vi "Get List of Names.vi"(8 "error in (no error)":errorcluster, 11 "Kasli in":refnum<class "Kasli.lvclass">) -> (0 "error out":errorcluster, 1 "List of IPs":string[](array[string]), 2 "List of Names":string[](array[string]), 3 "Kasli out":refnum<class "Kasli.lvclass">)   [LabVIEW 2020, in "Kasli Wrapper 2.0.lvlib" / "Kasli.lvclass"]
uses:
  Kasli.lvclass
  Kasli.lvclass/Kasli.ctl
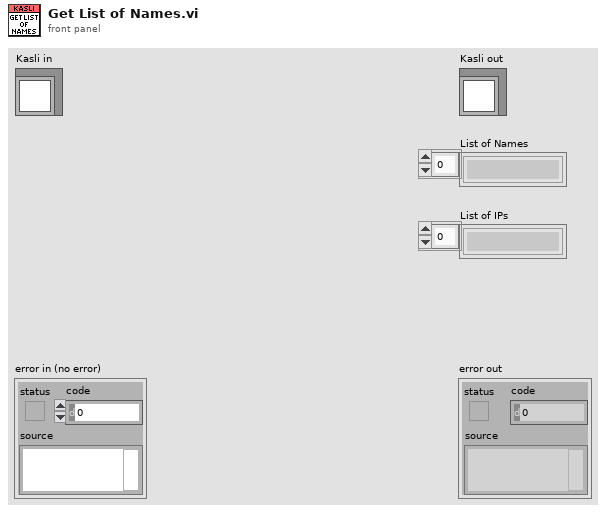
[diagram p1: front panel]
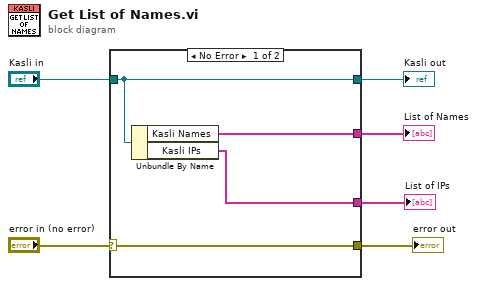
[diagram p0: block diagram]
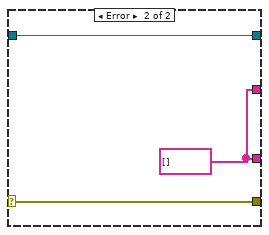
[diagram p2: hidden frame]
diagram:
  n1 = case shown="No Error" "error in (no error)" {
    selector: "error in (no error)" -> [w9 w12]
    tunnel: [w9 w12] -> w5
    tunnel: "Kasli in" -> [w10 w13]
    tunnel: [w10 w13] -> w3
    tunnel: [w8 w11] -> w2
    tunnel: [w7 w11] -> w1
    frame No Error {
      n2 = Unbundle By Name(w10) -> ("Kasli Names"=w8:string[], "Kasli IPs"=w7:string[])
    }
    frame Error {
      w11 = string[] []
    }
  }
  "error out" <- w5
  "Kasli out" <- w3
  "List of Names" <- w2
  "List of IPs" <- w1
